vi "configFilePractice.vi"() -> ()   [LabVIEW 2022 SP3]
uses:
  <vilib>/Utility/config.llb/Write Key (Boolean).vi
  <vilib>/Utility/config.llb/NI_LVConfig.lvlib
panel:
  in  "stop":bool
  out "found?":bool
  in  "configuration file path":path
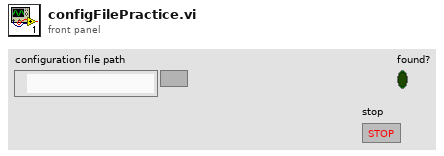
[diagram p1: front panel]
types:
  T1 = typedef "NI_LVConfig.lvlib/Config Data RefNum.ctl" = refnum<k1>
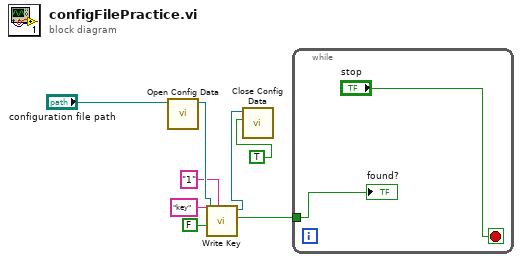
[diagram p0: block diagram]
diagram:
  n1 = call <vilib>:"Open Config Data.vi"("configuration file path"="configuration file path") -> ("refnum"=w6:T1)  [unwired: 8 in, 2 out]
  n2 = call-poly <vilib>:"Write Key.vi"("section"="1", "value"=FALSE, "key"="key", "refnum"=w6) -> ("found?"=w3:bool, "refnum out"=w2:T1)  [unwired: 5 in, 1 out]
  n3 = call <vilib>:"Close Config Data.vi"("write file if changed (T)"=TRUE, "refnum"=w2) -> ()  [unwired: 8 in, 2 out]
  n4 = while {
    tunnel: w3 -> [w10]
    stop <- "stop" stop-if-true
    "found?" <- w10
  }
